vi "PathPlanner_PathFinder_DoMajor.vi"   [LabVIEW 2019, in "PathPlanner24.lvlib"]
uses:
  PathPlanner24.lvlib
  PathPlanner_PathFinder_TopKey.vi
  PathPlanner_PathFinder_ComparePair.vi
  PathPlanner_GridPosition_HashCode.vi
  PathPlanner_PathFinder_UpdateState.vi
  PathPlanner_PathFinder_GetOpenNeighbors.vi
  PathPlanner_GridPosition_Equals.vi
  PathPlanner_PathFinder_IsWalkable.vi
  PathPlanner_PathFinder_GridPosToTranslation2d.vi
  <vilib>/Rock Robotics/WPI/ThirdParty/JAS_Junk/TrajLib/Translation2d_GetDistance.vi
  PathPlanner_PathFinder_Constants.vi
  <vilib>/Rock Robotics/WPI/ThirdParty/JAS_Junk/TrajLib/Translation2d_Create_DistAng.vi
  <vilib>/Rock Robotics/WPI/ThirdParty/JAS_Junk/TrajLib/Translation2d_Minus.vi
  <vilib>/Rock Robotics/WPI/ThirdParty/JAS_Junk/TrajLib/Translation2d_GetAngle.vi
  <vilib>/Rock Robotics/WPI/ThirdParty/JAS_Junk/TrajLib/Translation2d_Plus.vi
  PathPlanner_PathFinder_Heuristic.vi
  PathPlanner_GridPosition_Get.vi
  PathPlanner_PathFinder_Cost.vi
  PathPlanner_GridPosition_New.vi
  <vilib>/Rock Robotics/WPI/ThirdParty/JAS_Junk/TrajLib/Translation2d_Create.vi
  <vilib>/Rock Robotics/WPI/ThirdParty/JAS_Junk/TrajLib/Util_CalcDist.vi
  <vilib>/Rock Robotics/WPI/ThirdParty/JAS_Junk/TrajLib/Rotation2d_GetAngleCosSin.vi
  <vilib>/Rock Robotics/WPI/ThirdParty/JAS_Junk/TrajLib/Translation2d_GetXY.vi
  <vilib>/Rock Robotics/WPI/ThirdParty/JAS_Junk/TrajLib/Rotation2d_CreateXY.vi
  PathPlanner_PathFinder_IsCollision.vi
  PathPlanner_PathFinder_Globals.vi
  PathPlanner_PathFinder_ApplyControlSmooth.vi
  PathPlanner_PathFinder_ApplyAnchorSmooth.vi
  <vilib>/Utility/miscctls.llb/LVMapReplaceAction.ctl
types:
  T1 = typedef "LVMapReplaceAction.ctl" = enum32{"Modify Entry only if found", "Add or Modify Entry", "Delete Entry"}
  T2 = typedef "PathPlanner24.lvlib/PathPlannerFinderDoublePair.ctl" = cluster{"A":dbl, "B":dbl}
  T3 = typedef "PathPlanner24.lvlib/PathPlannerFinderGridPosition.ctl" = cluster{"X":i32, "Y":i32}
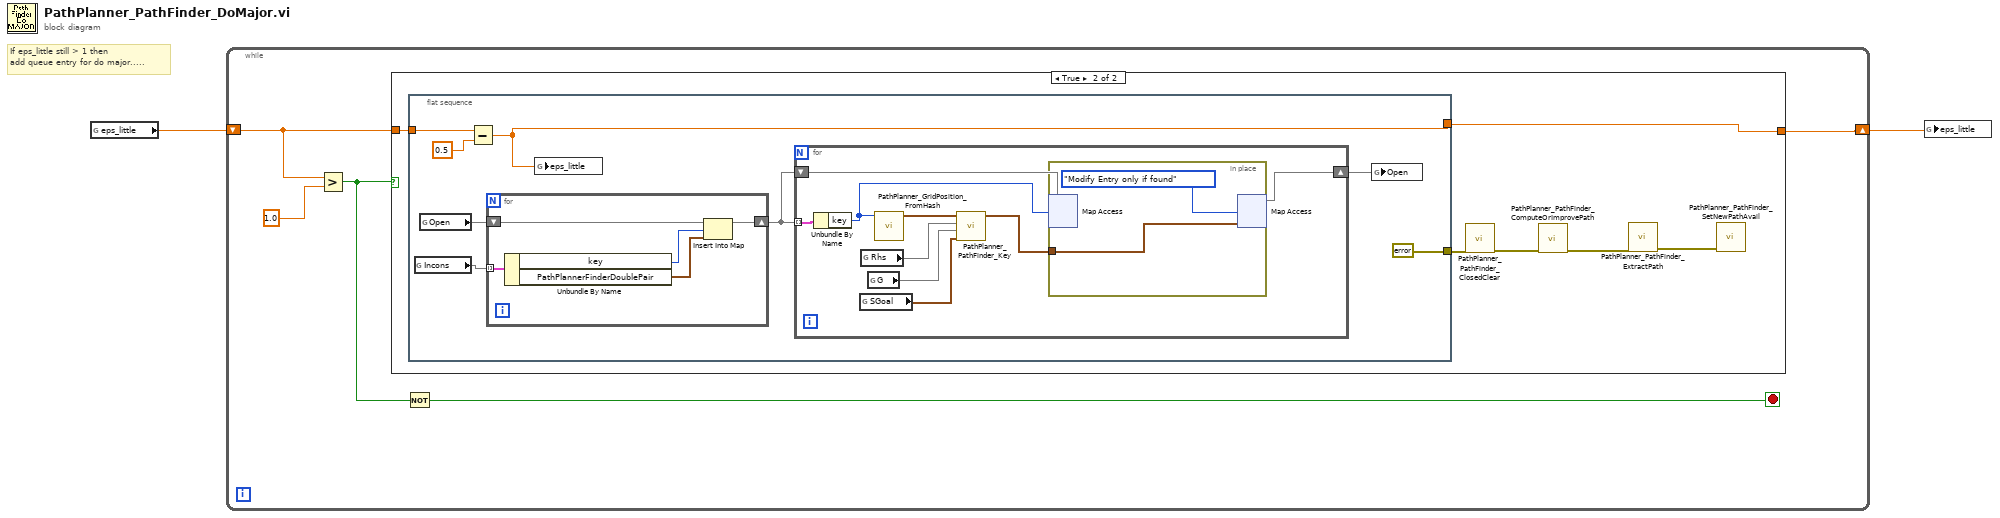
[diagram p0: block diagram]
diagram:
  # "If eps_little still > 1 then\nadd queue entry for do major....."
  n1 = global read "PathPlanner_PathFinder_Globals.vi" "eps_little"() -> (w2:dbl)
  n2 = while {
    shift-right: [w5] -> w1
    shift-left: w2 -> [w6]
    stop <- w3 stop-if-true
    n3 = Greater?(x=w6, y=1.0) -> (0:w4:bool)
    n4 = case shown="True" w4 {
      tunnel: w6 -> [w8 w14]
      tunnel: [w8 w10] -> w5
      frame False {
      }
      frame True {
        n5 = flat-sequence {
          tunnel: w14 -> [w22]
          tunnel: [w16] -> w10
          tunnel: [errorcluster {"status"=FALSE, "code"=0, "source"=""} ("error in (no error)")] -> w9
          frame #0 {
            n6 = global read "PathPlanner_PathFinder_Globals.vi" "Incons"() -> (w20:map{i32, T2})
            n7 = global read "PathPlanner_PathFinder_Globals.vi" "Open"() -> (w19:map{i32, T2})
            n8 = Subtract(x=w22, y=0.5) -> (x-y=w16:dbl)
            n9 = for {
              tunnel: w20 -> [w37] mode=indexing
              shift-right: [w36] -> w18
              shift-left: w19 -> [w38]
              n10 = Unbundle By Name(w37) -> ("key"=w35:i32, "PathPlannerFinderDoublePair"=w34:T2)
              n11 = Insert Into Map(map in=w38, key=w35, value=w34) -> (map out=w36:map{i32, T2})  [unwired: 2 out]
            }
            n12 = global write "PathPlanner_PathFinder_Globals.vi" "eps_little"(w16) -> ()
            n13 = for {
              tunnel: w18 -> [w30] mode=indexing
              shift-right: [w23] -> w17
              shift-left: w18 -> [w26]
              n14 = Unbundle By Name(w30) -> ("key"=w24:i32)
              n15 = global read "PathPlanner_PathFinder_Globals.vi" "SGoal"() -> (w27:T3)
              n16 = global read "PathPlanner_PathFinder_Globals.vi" "Rhs"() -> (w29:map{i32, dbl})
              n17 = global read "PathPlanner_PathFinder_Globals.vi" "G"() -> (w28:map{i32, dbl})
              n18 = call "PathPlanner_GridPosition_FromHash.vi"("Hash"=w24) -> ("GridPosition"=w31:T3)  [unwired: 10 in]
              n19 = call "PathPlanner_PathFinder_Key.vi"("Sstart"=w27, "G"=w28, "RHS"=w29, "S"=w31) -> ("DoublePair"=w25:T2)  [unwired: 7 in]
              n20 = in-place {
                in-place-border: w25 -> [w32]
                n21 = in-place-map #1(w26, w24) -> ()  [unwired: 1 in, 2 out]
                n22 = in-place-map #1(w32, LVMapReplaceAction."Modify Entry only if found" ("action")) -> (w23:map{i32, T2})  [unwired: 2 out]
              }
            }
            n23 = global write "PathPlanner_PathFinder_Globals.vi" "Open"(w17) -> ()
          }
        }
        n24 = call "PathPlanner_PathFinder_ClosedClear.vi"("error in (no error)"=w9) -> ("error out"=w11:errorcluster)  [unwired: 10 in]
        n25 = call "PathPlanner_PathFinder_ComputeOrImprovePath.vi"("error in (no error)"=w11) -> ("error out"=w12:errorcluster)  [unwired: 10 in]
        n26 = call "PathPlanner_PathFinder_ExtractPath.vi"("error in (no error)"=w12) -> ("error out"=w13:errorcluster)  [unwired: 10 in]
        n27 = call "PathPlanner_PathFinder_SetNewPathAvail.vi"("error in (no error)"=w13) -> ()  [unwired: 10 in, 1 out]
      }
    }
    n28 = Not(x=w4) -> (.not. x?=w3:bool)
  }
  n29 = global write "PathPlanner_PathFinder_Globals.vi" "eps_little"(w1) -> ()
